vi "Util_Trajectory_WriteFile_PathFinder.vi"(6 "Trajectory Is Relative":bool, 7 "UTIL_PATHFINDER_CONFIG":T7 {"ActualMaxVelocity-inches per sec" format="%21.5f"; "WheelbaseDepth-inches" format="%21.5f"; "WheelbaseWidth-inches" format="%21.5f"; "TimeDelta-Seconds" format="%21.5f"; "MaxJerk--Inches per sec2" format="%21.5f"; "MaxAcceleration - inches per sec2" format="%21.5f"; "PathMaxVelocity - inches per sec" format="%21.5f"}, 8 "UtilityWayPoints":T6[](array[typedef]) {"ANGLE" format="%13.3f"; "Y" format="%13.3f"; "X" format="%13.3f"}, 9 "TRAJECTORY":T1 {"TotalTImeSecs" format="%20.3f"}, 10 "Comment":string, 11 "Trajectory File Name":path) -> (0 "error out":errorcluster)   [LabVIEW 2019, in "Trajectory_Library.lvlib"]
doc: "Create a CSV file from a Trajectory data structure. This can be used on a PC or the RoboRIO. This is a customized version for Pathfinder created trajectories.\n\nParameters:\n - Trajectory - Data structure containing trajectory\n - PathfinderConfig - Data structure with pathfinder configuration.\n - Trajectory File Name - File name to write to. Existing files are overwritten.\n - Comment - Comment string to include in file comments.\n - Waypoints - waypoints to include in file comments\n - TrajectoryIsRelative - Relative if TRUE otherwise absolute.\n\nReturns:\n - Error out - returned error cluster"
uses:
  Trajectory_Library.lvlib
  UTIL_PATHFINDER_CONFIG.ctl
  UTIL_WAYPOINT.ctl
  TRAJECTORY.ctl
  TRAJ_STATE.ctl
  POSE2D.ctl
  TRANSLATION2D.ctl
  ROTATION2D.ctl
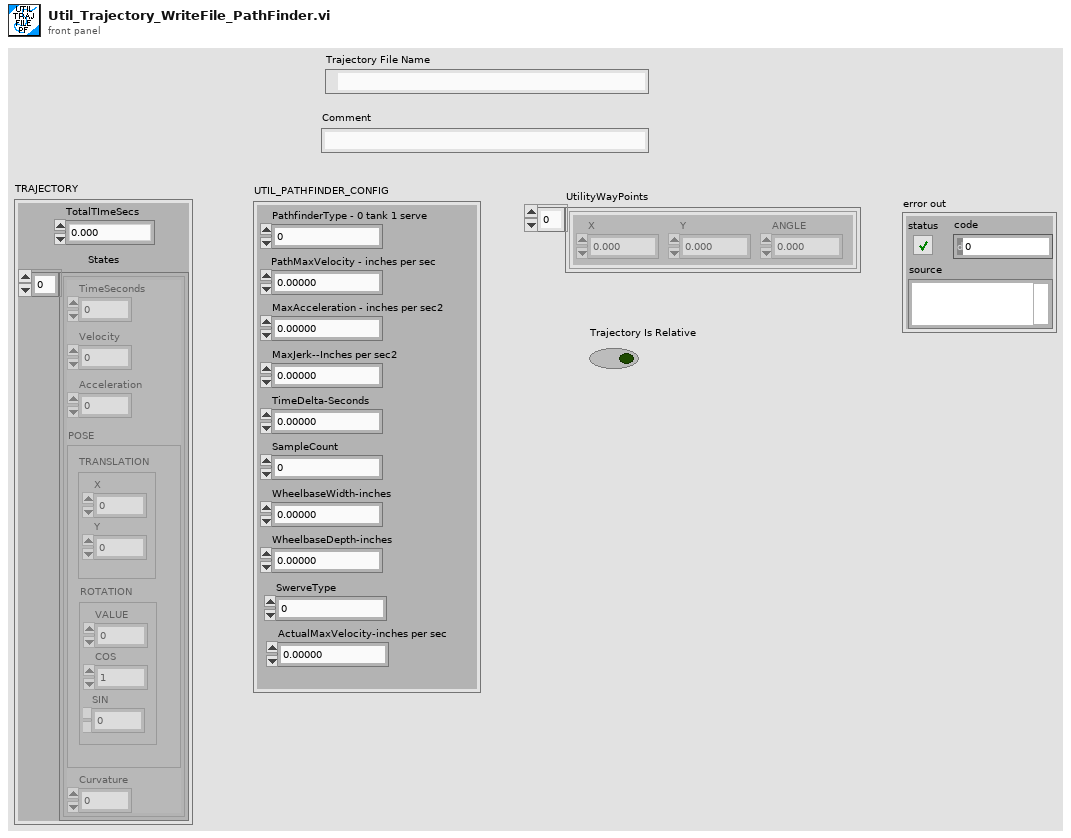
[diagram p1: front panel]
types:
  T1 = typedef "Trajectory_Library.lvlib/TRAJECTORY.ctl" = cluster{"TotalTImeSecs":dbl, "States":T2[]}
  T2 = typedef "Trajectory_Library.lvlib/TRAJ_STATE.ctl" = cluster{"TimeSeconds":dbl, "Velocity":dbl, "Acceleration":dbl, "POSE":T3, "Curvature":dbl}
  T3 = typedef "Trajectory_Library.lvlib/POSE2D.ctl" = cluster{"TRANSLATION":T4, "ROTATION":T5}
  T4 = typedef "Trajectory_Library.lvlib/TRANSLATION2D.ctl" = cluster{"X":dbl, "Y":dbl}
  T5 = typedef "Trajectory_Library.lvlib/ROTATION2D.ctl" = cluster{"VALUE":dbl, "COS":dbl, "SIN":dbl}
  T6 = typedef "Trajectory_Library.lvlib/UTIL_WAYPOINT.ctl" = cluster{"X":dbl, "Y":dbl, "ANGLE":dbl}
  T7 = typedef "Trajectory_Library.lvlib/UTIL_PATHFINDER_CONFIG.ctl" = cluster{"PathfinderType - 0 tank 1 serve":i32, "PathMaxVelocity - inches per sec":dbl, "MaxAcceleration - inches per sec2":dbl, "MaxJerk--Inches per sec2":dbl, "TimeDelta-Seconds":dbl, "SampleCount":i32, "WheelbaseWidth-inches":dbl, "WheelbaseDepth-inches":dbl, "SwerveType":i32, "ActualMaxVelocity-inches per sec":dbl}
  T8 = enum16{"open", "replace", "create", "open or create", "replace or create", "replace or create with confirmation"}
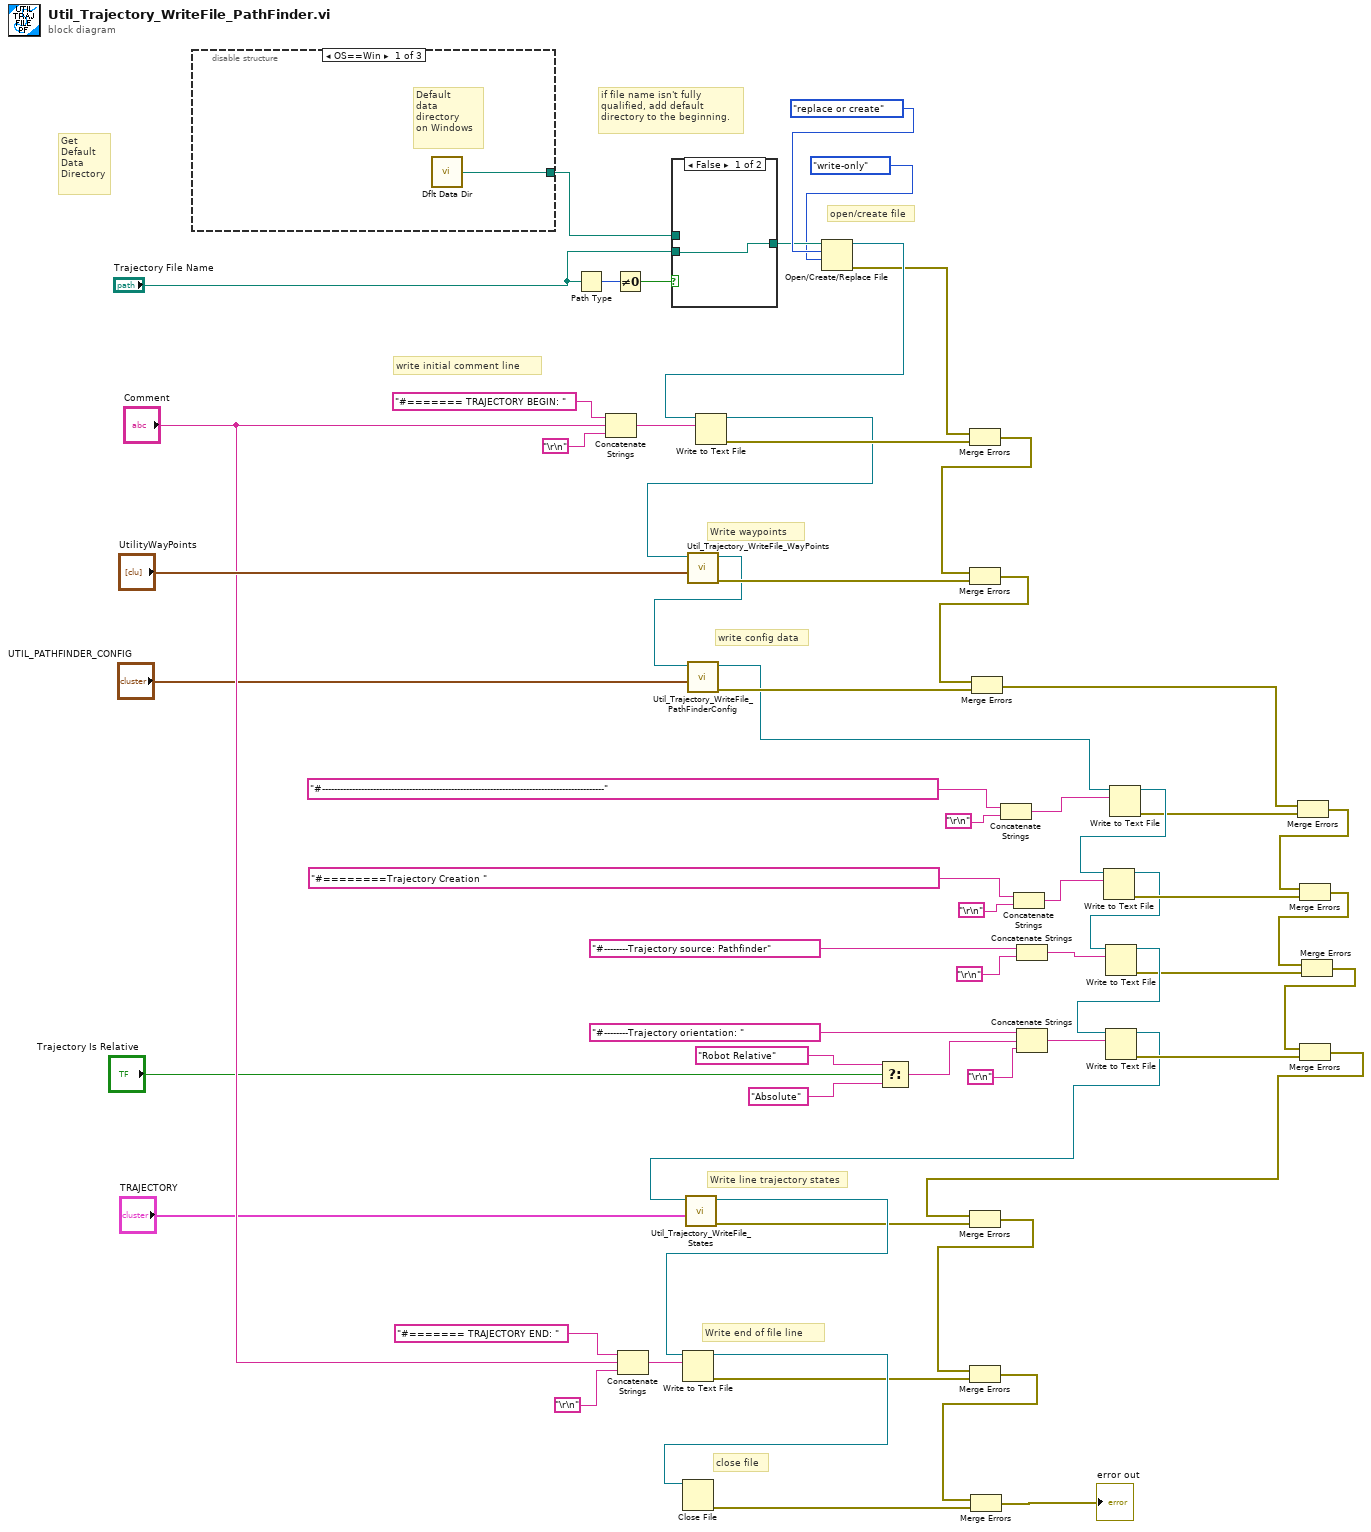
[diagram p0: block diagram]
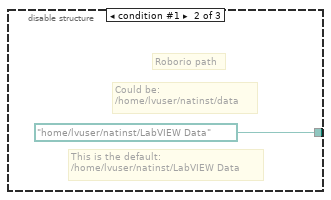
[diagram p2: hidden frame]
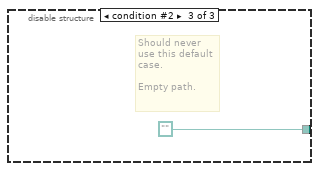
[diagram p3: hidden frame]
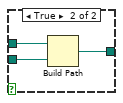
[diagram p4: hidden frame]
diagram:
  # "write config data"
  # "Write line trajectory states"
  # "open/create file"
  # "if file name isn't fully \nqualified, add default\ndirectory to the beginning."
  # "Get\nDefault\nData\nDirectory"
  # "Write waypoints"
  # "close file"
  # "Write end of file line"
  # "write initial comment line"
  n1 = disable-structure shown="OS==Win" {
    disable-tunnel: [w65 path "/home/lvuser/natinst/LabVIEW Data" path ""] -> w54
    frame condition #0 (active) {
      # "Default\ndata\ndirectory\non Windows"
      n2 = call <vilib>:"Dflt Data Dir.vi"() -> ("App:Default Data Directory"=w65:path)
    }
    frame condition #1 {
      # "This is the default:\n/home/lvuser/natinst/LabVIEW Data"
      # "Could be:\n/home/lvuser/natinst/data"
      # "Roborio path"
    }
    frame condition #2 {
      # "Should never\nuse this default\ncase.\n\nEmpty path."
    }
  }
  n3 = Path Type(1:"Trajectory File Name") -> (0:w57:i16)
  n4 = Concatenate Strings("#======= TRAJECTORY BEGIN: " ("string"), "Comment", "\r\n") -> (w62:string)
  n5 = Not Equal To 0?(x=w57) -> (x != 0?=w56:bool)
  n6 = Concatenate Strings("#======= TRAJECTORY END: " ("string"), "Comment", "\r\n") -> (w58:string)
  n7 = case shown="False" w56 {
    tunnel: [w68 w71] -> w53
    tunnel: w54 -> [_ w70]
    tunnel: "Trajectory File Name" -> [w68 w69]
    frame False {
    }
    frame True {
      n8 = Build Path(base path=w70, name or relative path=w69) -> (appended path=w71:path)
    }
  }
  n9 = Open/Create/Replace File(file path (use dialog)=w53, operation (0:open)=T8."replace or create", access (0:read/write)=enum16{"read/write", "read-only", "write-only"}."write-only") -> (refnum out=w50:refnum<file>, error out=w45:errorcluster)  [unwired: 3 in, 1 out]
  n10 = Write to Text File(file (use dialog)=w50, text=w62) -> (refnum out=w36:refnum<file>, error out=w46:errorcluster)  [unwired: 2 in, 1 out]
  n11 = call "Util_Trajectory_WriteFile_WayPoints.vi"("UtilityWayPoints"="UtilityWayPoints", "Byte Steam File In"=w36) -> ("error out"=w44:errorcluster, "Byte Steam File Out"=w35:refnum<file>)  [unwired: 8 in]
  n12 = call "Util_Trajectory_WriteFile_PathFinderConfig.vi"("UTIL_PATHFINDER_CONFIG"="UTIL_PATHFINDER_CONFIG", "Byte Steam File In"=w35) -> ("error out"=w34:errorcluster, "Byte Steam File Out"=w15:refnum<file>)  [unwired: 8 in]
  n13 = Select(t="Robot Relative" ("string"), s="Trajectory Is Relative", f="Absolute" ("string")) -> (s? t:f=w23:string)
  n14 = Merge Errors(w45, w46) -> (w37:errorcluster)
  n15 = Merge Errors(w37, w44) -> (w33:errorcluster)
  n16 = Merge Errors(w33, w34) -> (w12:errorcluster)
  n17 = Concatenate Strings("#----------------------------------------------------------------------------------------------" ("string"), "\r\n") -> (w27:string)
  n18 = Concatenate Strings("#========Trajectory Creation " ("string"), "\r\n") -> (w30:string)
  n19 = Concatenate Strings("#--------Trajectory source: Pathfinder" ("string"), "\r\n") -> (w10:string)
  n20 = Concatenate Strings("#--------Trajectory orientation: " ("string"), w23, "\r\n") -> (w25:string)
  n21 = Write to Text File(file (use dialog)=w15, text=w27) -> (refnum out=w19:refnum<file>, error out=w17:errorcluster)  [unwired: 2 in, 1 out]
  n22 = Write to Text File(file (use dialog)=w19, text=w30) -> (refnum out=w7:refnum<file>, error out=w18:errorcluster)  [unwired: 2 in, 1 out]
  n23 = Write to Text File(file (use dialog)=w7, text=w10) -> (refnum out=w6:refnum<file>, error out=w5:errorcluster)  [unwired: 2 in, 1 out]
  n24 = Write to Text File(file (use dialog)=w6, text=w25) -> (refnum out=w14:refnum<file>, error out=w24:errorcluster)  [unwired: 2 in, 1 out]
  n25 = call "Util_Trajectory_WriteFile_States.vi"("Trajectory"="TRAJECTORY", "Byte Steam File In"=w14) -> ("error out"=w43:errorcluster, "Byte Steam File Out"=w48:refnum<file>)  [unwired: 8 in]
  n26 = Write to Text File(file (use dialog)=w48, text=w58) -> (refnum out=w47:refnum<file>, error out=w41:errorcluster)  [unwired: 2 in, 1 out]
  n27 = Close File(refnum=w47) -> (error out=w40:errorcluster)  [unwired: 1 in, 1 out]
  n28 = Merge Errors(w12, w17) -> (w16:errorcluster)
  n29 = Merge Errors(w16, w18) -> (w4:errorcluster)
  n30 = Merge Errors(w4, w5) -> (w3:errorcluster)
  n31 = Merge Errors(w3, w24) -> (w11:errorcluster)
  n32 = Merge Errors(w11, w43) -> (w42:errorcluster)
  n33 = Merge Errors(w42, w41) -> (w39:errorcluster)
  n34 = Merge Errors(w39, w40) -> (→"error out":errorcluster)
